vi "EnqueueMessage.vi"(6 "Priority Message? (F)":bool, 8 "error in (no error)":errorcluster, 9 "MessageData":variant, 10 "Message":string, 11 "MessageQueue":refnum<queue>) -> (0 "error out":errorcluster, 3 "dupMessageQueue":refnum<queue>)   [LabVIEW 2015]
doc: "Reiht eine Nachricht ans Ende oder an den Anfang der Queue."
uses:
  TypeDefs/MessageCluster.ctl
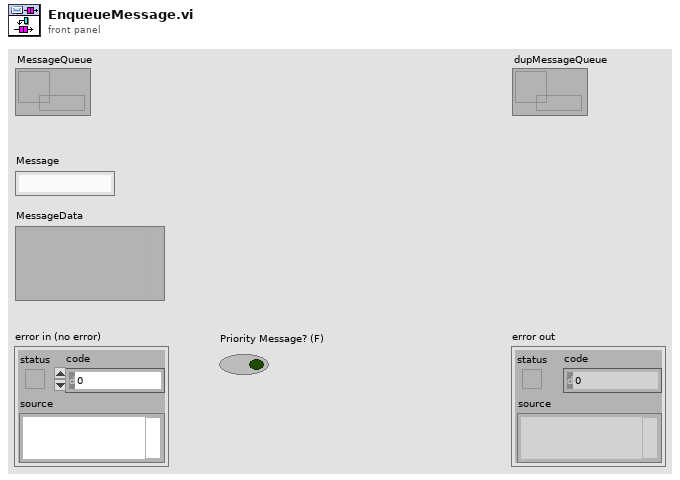
[diagram p1: front panel]
types:
  T1 = typedef "MessageCluster.ctl" = cluster{"Message":string, "MessageData":variant}
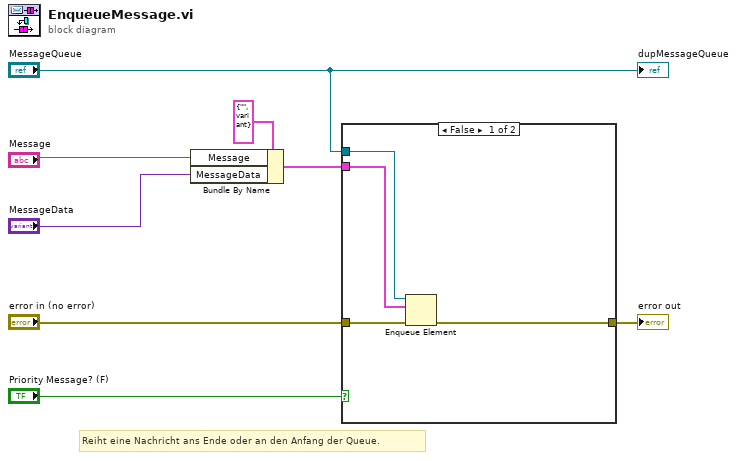
[diagram p0: block diagram]
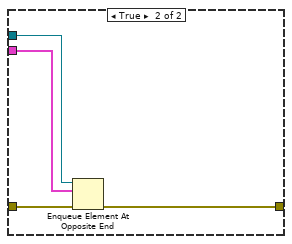
[diagram p2: hidden frame]
diagram:
  # "Reiht eine Nachricht ans Ende oder an den Anfang der Queue."
  n1 = Bundle By Name(cluster=T1 {"Message"="", "MessageData"=variant} ("Message Cluster"), "Message"="Message", "MessageData"="MessageData") -> (w1:T1)
  n2 = case shown="False" "Priority Message? (F)" {
    tunnel: "error in (no error)" -> [w12 w16]
    tunnel: [w11 w15] -> w3
    tunnel: "MessageQueue" -> [w10 w14]
    tunnel: w1 -> [w9 w13]
    frame False {
      n3 = Enqueue Element(queue=w10, element=w9, error in (no error)=w12) -> (error out=w11:errorcluster)  [unwired: 1 in, 2 out]
    }
    frame True {
      n4 = Enqueue Element At Opposite End(queue=w14, element=w13, error in (no error)=w16) -> (error out=w15:errorcluster)  [unwired: 1 in, 2 out]
    }
  }
  "error out" <- w3
  "dupMessageQueue" <- "MessageQueue"
